vi "CreateProtectedEvents.vi"(8 "error in (no error)":errorcluster, 11 "Measurement":refnum<class "Measurement.lvclass">) -> (0 "error out":errorcluster, 3 "Measurement out":refnum<class "Measurement.lvclass">)   [LabVIEW 2017, in "Measurement.lvclass"]
doc: "JKI State Machine Objects (SMO) 1.3.0.56\nJKI - JKI\nCopyright (c) 2017, JKI"
uses:
  Measurement.lvclass
  Measurement.lvclass/Measurement.ctl
  Typedefs/ProtectedEvents--Measurement.Begin.ctl
  Typedefs/ProtectedEvents--Measurement.Pause.ctl
  Typedefs/ProtectedEvents--Measurement.End.ctl
  Typedefs/ProtectedEvents--Measurement.Initialize.ctl
  Typedefs/ProtectedEvents--Measurement.Uninitialize.ctl
  <vilib>/JKI/JKI SMO/SMO/SMO.lvclass
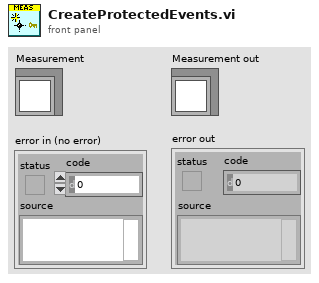
[diagram p1: front panel]
types:
  T1 = typedef "Measurement.lvclass/PrivateData--Ref.ctl" = refnum<data-value>
  T2 = typedef "Measurement.lvclass/ProtectedEvents--Measurement.Uninitialize.ctl" = bool
  T3 = typedef "Measurement.lvclass/ProtectedEvents--Measurement.Initialize.ctl" = bool
  T4 = typedef "Measurement.lvclass/ProtectedEvents--Measurement.End.ctl" = bool
  T5 = typedef "Measurement.lvclass/ProtectedEvents--Measurement.Pause.ctl" = bool
  T6 = typedef "Measurement.lvclass/ProtectedEvents--Measurement.Begin.ctl" = bool
  T7 = typedef "Measurement.lvclass/PrivateData--Cluster.ctl" = cluster{"Public Events":T8, "Protected Events":T9}
  T8 = typedef "Measurement.lvclass/PublicEvents--Cluster.ctl" = cluster{"Initialized":refnum<user-event>, "Measured":refnum<user-event>, "Finished":refnum<user-event>, "Uninitialized":refnum<user-event>}
  T9 = typedef "Measurement.lvclass/ProtectedEvents--Cluster.ctl" = cluster{"Initialize":refnum<user-event>, "Begin":refnum<user-event>, "Pause":refnum<user-event>, "End":refnum<user-event>, "Uninitialize":refnum<user-event>}
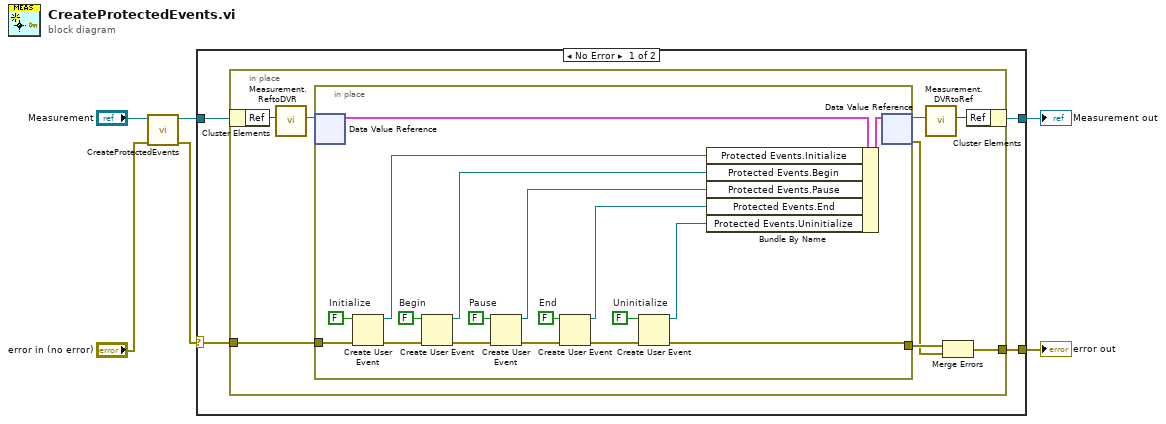
[diagram p0: block diagram]
diagram:
  n1 = call-parent "CreateProtectedEvents.vi"("error in (no error)"="error in (no error)", "SMO"="Measurement") -> ("error out"=w3:errorcluster, "SMO out"=w4:refnum<class "Measurement.lvclass">)  [unwired: 8 in]
  n2 = case shown="No Error" w3 {
    selector: w3 -> [w9 w37]
    tunnel: w4 -> [w10 w38]
    tunnel: [w8 w37] -> w1
    tunnel: [w7 w38] -> w2
    frame No Error {
      n3 = in-place {
        in-place-border: w9 -> [w14]
        in-place-border: [w11] -> w8
        n4 = in-place-cluster #1(w10) -> ("Ref"=w18:u32)
        n5 = call "Measurement.ReftoDVR.vi"("Ref"=w18) -> ("Ref"=w17:T1)  [unwired: 10 in]
        n6 = in-place {
          in-place-border: w14 -> [w34]
          in-place-border: [w21] -> w13
          w20 = T2 FALSE  # Uninitialize
          w23 = T3 FALSE  # Initialize
          w26 = T4 FALSE  # End
          w27 = T5 FALSE  # Pause
          w31 = T6 FALSE  # Begin
          n7 = in-place-dvr #2(w17) -> (w36:T7)  [unwired: 1 out]
          n8 = Create User Event(user event datatype=w23, error in=w34) -> (user event=w33:refnum<user-event>, error out=w32:errorcluster)
          n9 = Create User Event(user event datatype=w31, error in=w32) -> (user event=w30:refnum<user-event>, error out=w29:errorcluster)
          n10 = Create User Event(user event datatype=w27, error in=w29) -> (user event=w25:refnum<user-event>, error out=w28:errorcluster)
          n11 = Create User Event(user event datatype=w26, error in=w28) -> (user event=w24:refnum<user-event>, error out=w22:errorcluster)
          n12 = Create User Event(user event datatype=w20, error in=w22) -> (user event=w19:refnum<user-event>, error out=w21:errorcluster)
          n13 = Bundle By Name(cluster=w36, "Protected Events.Initialize"=w33, "Protected Events.Begin"=w30, "Protected Events.Pause"=w25, "Protected Events.End"=w24, "Protected Events.Uninitialize"=w19) -> (w35:T7)
          n14 = in-place-dvr #2(w35) -> (w16:T1, w12:errorcluster)
        }
        n15 = call "Measurement.DVRtoRef.vi"("Ref"=w16) -> ("Ref"=w15:u32)  [unwired: 10 in]
        n16 = Merge Errors(w13, w12) -> (w11:errorcluster)
        n17 = in-place-cluster #1("Ref"=w15) -> (w7:refnum<class "Measurement.lvclass">)
      }
    }
    frame Error {
    }
  }
  "error out" <- w1
  "Measurement out" <- w2
